vi "lijnvolgen.vi"() -> ()   [LabVIEW 2019]
uses:
  <vilib>/myRIO/Instrument Drivers/Onboard IO/AI/typedefs/AI Reference.ctl
  <vilib>/myRIO/Common/Instrument Driver Framework/Utilities/typedefs/myRIO Generic Hardware Reference.ctl
  <vilib>/myRIO/Common/Instrument Driver Framework/Utilities/typedefs/Hardware Version Enum.ctl
  <vilib>/myRIO/Common/Instrument Driver Framework/Utilities/typedefs/myRIO v1.0 Reference.ctl
  <vilib>/myRIO/Common/Instrument Driver Framework/Utilities/typedefs/Generic FPGA Reference.ctl
  <vilib>/myRIO/Common/Instrument Driver Framework/myRIO v1.0/AI/typedefs/AI Channels List.ctl
  <vilib>/myRIO/Common/Instrument Driver Framework/myRIO v1.0/AI/typedefs/AI Channels Enum.ctl
  <vilib>/myRIO/Common/Instrument Driver Framework/Utilities/typedefs/Analog Scaling Constants List.ctl
  <vilib>/myRIO/Common/Instrument Driver Framework/Utilities/typedefs/Analog Scaling Constants.ctl
  <vilib>/userDefined/High Color/nirio_resource_hc.ctl
  <vilib>/myRIO/Instrument Drivers/Onboard IO/AO/typedefs/AO Reference.ctl
  <vilib>/myRIO/Common/Instrument Driver Framework/myRIO v1.0/AO/typedefs/AO Channels List.ctl
  <vilib>/myRIO/Common/Instrument Driver Framework/myRIO v1.0/AO/typedefs/AO Channels Enum.ctl
  <vilib>/myRIO/Common/Instrument Driver Framework/Utilities/vis/Is FPGA Ref Available.vi
  <vilib>/myRIO/Common/Instrument Driver Framework/myRIO v1.0/AI/vis/myRIO v1.1 Open AI.vi
  <vilib>/myRIO/Instrument Drivers/Onboard IO/AI/vis/Read.vi
  <vilib>/myRIO/Common/Instrument Driver Framework/myRIO v1.0/AO/vis/myRIO v1.1 Open AO.vi
  <vilib>/myRIO/Instrument Drivers/Onboard IO/AO/vis/Write.vi
  <vilib>/myRIO/Common/Instrument Driver Framework/Utilities/vis/Validate Channels.vi
  <vilib>/myRIO/Common/Instrument Driver Framework/myRIO v1.0/AI/vis/myRIO v1.0 Reserve AI.vi
  <vilib>/myRIO/Common/Instrument Driver Framework/myRIO v1.0/AO/vis/myRIO v1.0 Reserve AO.vi
  <vilib>/myRIO/Common/Instrument Driver Framework/myRIO v1.0/AI/vis/myRIO v1.0 Build MUX Configuration AI.vi
  <vilib>/myRIO/Common/Instrument Driver Framework/myRIO v1.0/Resource Manager/vis/myRIO v1.0 Reserve Channel List.vi
  <vilib>/myRIO/Common/Instrument Driver Framework/myRIO v1.0/AO/vis/myRIO v1.0 Build MUX Configuration AO.vi
  <vilib>/myRIO/Common/Instrument Driver Framework/myRIO v1.0/Resource Manager/vis/myRIO v1.0 Reserve Channel.vi
  <vilib>/myRIO/Common/Instrument Driver Framework/myRIO v1.0/Resource Manager/vis/myRIO v1.0 Unreserve Channel.vi
  <vilib>/myRIO/Common/Instrument Driver Framework/myRIO v1.0/Resource Manager/vis/myRIO v1.0 Build Mutex Name.vi
  <vilib>/Utility/VariantDataType/GetNumericInfo.vi
  <vilib>/Utility/error.llb/Error Cluster From Error Code.vi
  <vilib>/myRIO/Common/Instrument Driver Framework/myRIO v1.0/myRIO v1.1 Open.vi
  <vilib>/myRIO/Common/Instrument Driver Framework/myRIO v1.0/AI/vis/myRIO v1.0 Get Scaling Constants AI.vi
  <vilib>/myRIO/Common/Instrument Driver Framework/Utilities/vis/IO Manager.vi
  <vilib>/myRIO/Common/Instrument Driver Framework/Utilities/vis/Configuration Manager.vi
  <vilib>/myRIO/Common/Instrument Driver Framework/myRIO v1.0/myRIO v1.0 Close.vi
  <vilib>/myRIO/Common/Instrument Driver Framework/myRIO v1.0/AI/vis/myRIO v1.0 Read AI.vi
  <vilib>/myRIO/Common/Instrument Driver Framework/myRIO v1.0/AO/vis/myRIO v1.0 Get Scaling Constants AO.vi
  <vilib>/myRIO/Common/Instrument Driver Framework/myRIO v1.0/AO/vis/myRIO v1.0 Write AO.vi
  <vilib>/myRIO/Express VI/Onboard IO/AI/AI Express VI.xnode
  <vilib>/myRIO/Instrument Drivers/Onboard IO/AI/vis/myRIO AI Open.xnode
  <vilib>/myRIO/Express VI/Onboard IO/AO/AO Express VI.xnode
  <vilib>/myRIO/Instrument Drivers/Onboard IO/AO/vis/myRIO AO Open.xnode
  <vilib>/myRIO/Instrument Drivers/Onboard IO/AO/AO.lvlib
  <vilib>/myRIO/Instrument Drivers/Onboard IO/AI/AI.lvlib
panel:
  in  "Boolean":bool
  out "Numeric 4":i32
  out "analoog":dbl[](array[numeric])
  out "Array 3":i32[](array[numeric])
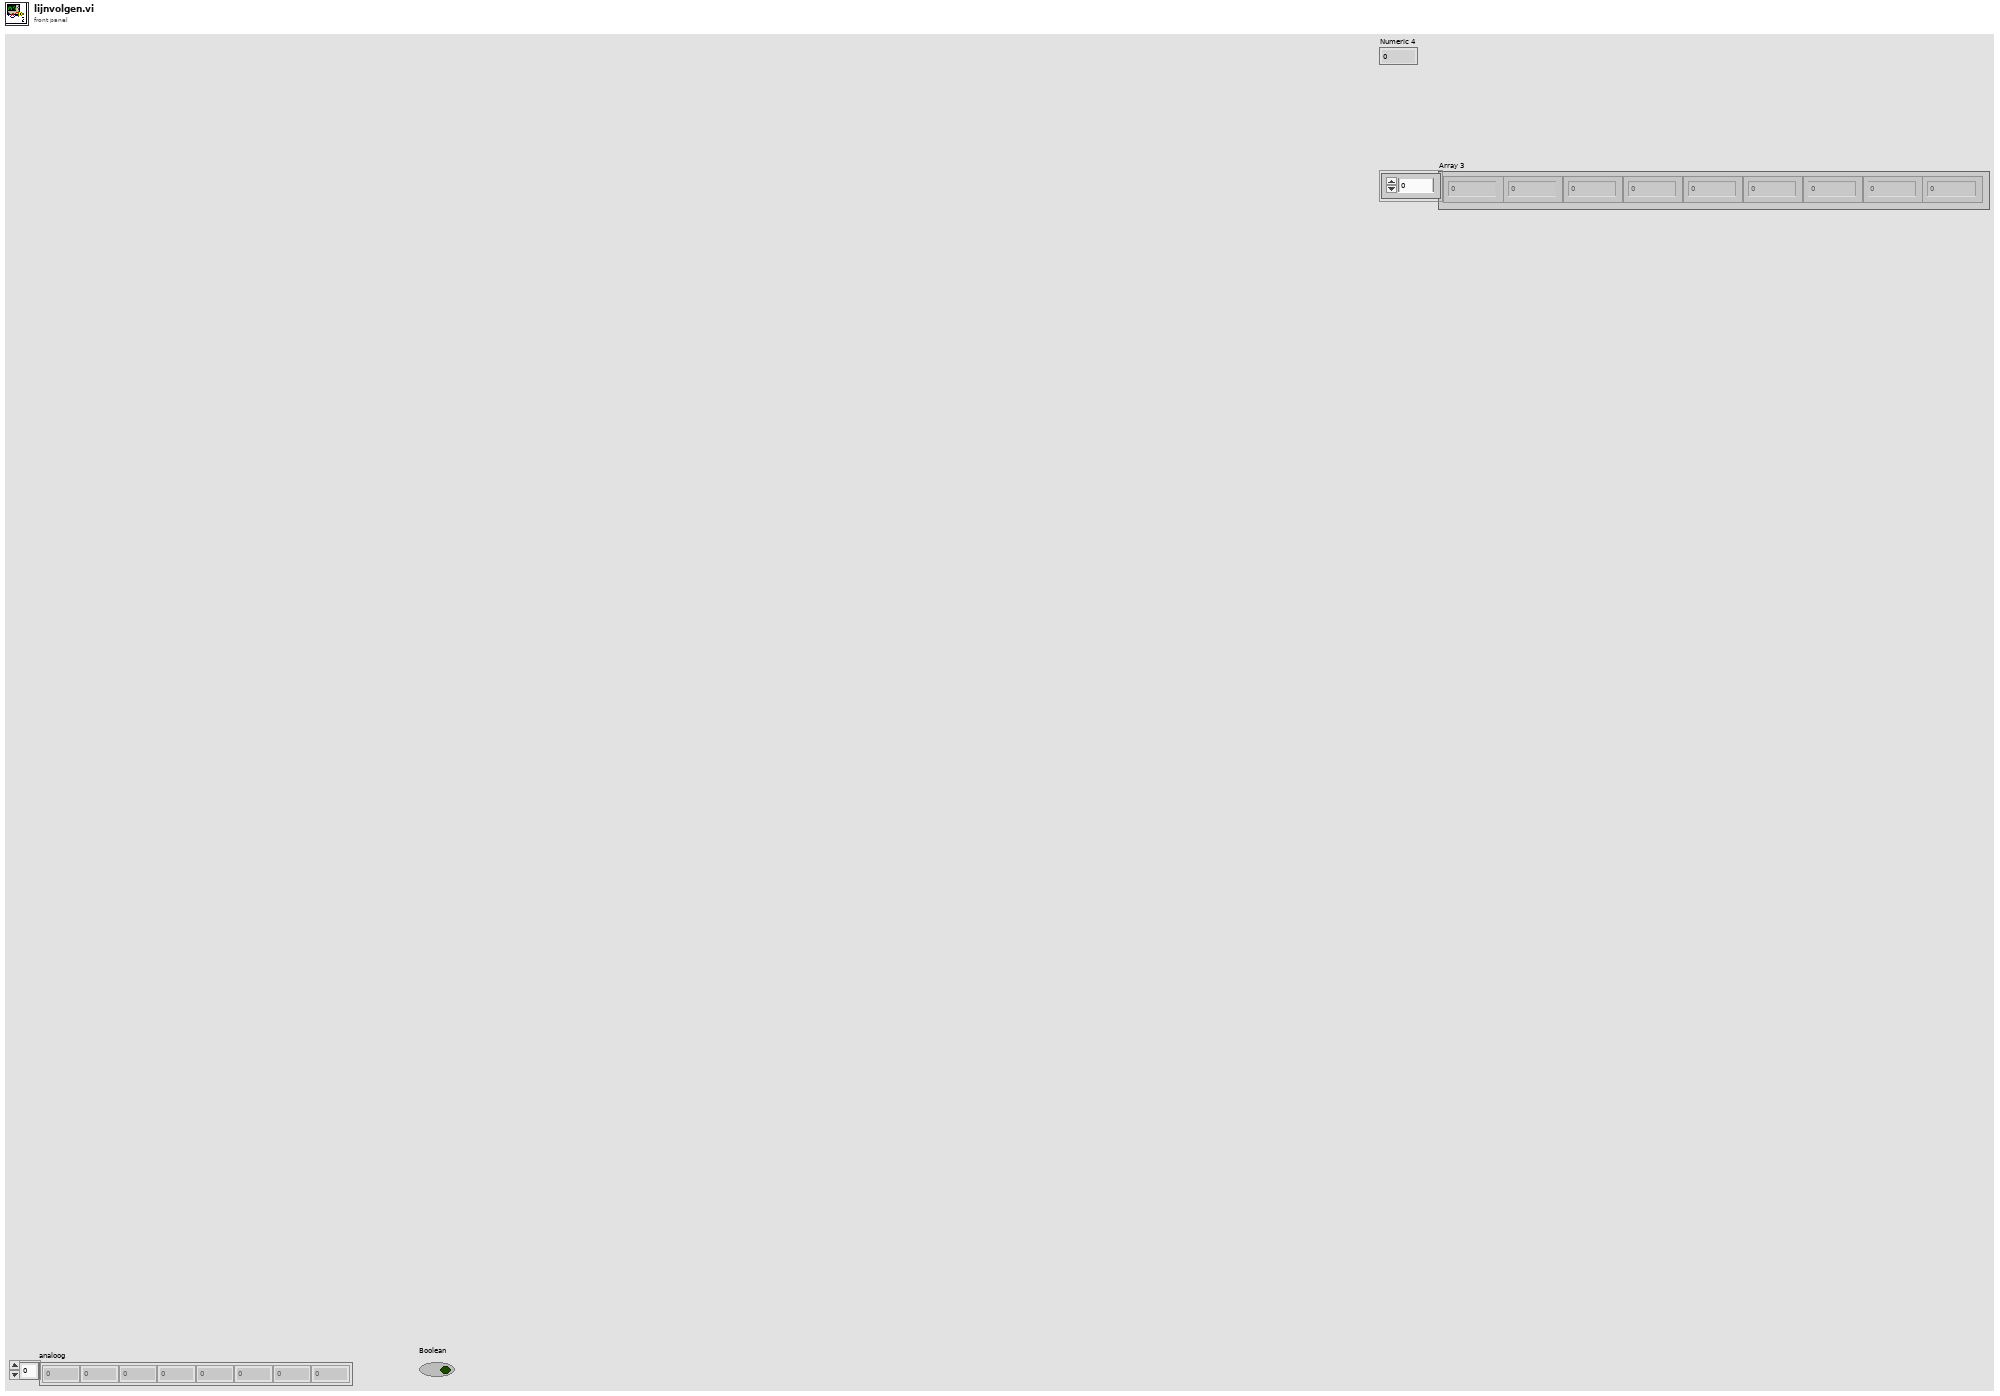
[diagram p1: front panel]
types:
  T1 = typedef "AO.lvlib/AO Reference.ctl" = cluster{"myRIO Reference":T2, "AO Channel List":T6, "AO Scaling Constant List":T8}
  T2 = typedef "myRIO Generic Hardware Reference.ctl" = cluster{"myRIO Model":T3, "myRIO Hardware Reference":T4}
  T3 = typedef "Hardware Version Enum.ctl" = enum16{"Unknown", "myRIO-1900", "myRIO-1950", "roboRIO", "NI ELVIS RIO CM", "ELVIS III"}
  T4 = typedef "myRIO v1.0 Reference.ctl" = cluster{"Generic FPGA Reference":T5, "Allow multiple opens":bool}
  T5 = typedef "Generic FPGA Reference.ctl" = refnum<k20>
  T6 = typedef "AO Channels List.ctl" = T7[]
  T7 = typedef "AO Channels Enum.ctl" = enum16{"Not Connected", "AudioOut/Left", "AudioOut/Right", "C/AO0", "C/AO1", "A/AO0", "A/AO1", "B/AO0", "B/AO1"}
  T8 = typedef "Analog Scaling Constants List.ctl" = T9[]
  T9 = typedef "Analog Scaling Constants.ctl" = cluster{"LSB Weight (Volts)":dbl, "Offset (Volts)":dbl, "Signed?":bool}
  T10 = typedef "nirio_resource_hc.ctl" = tag
  T11 = typedef "AI.lvlib/AI Reference.ctl" = cluster{"myRIO Reference":T2, "AI Channels List":T12, "AI Scaling Constants List":T8}
  T12 = typedef "AI Channels List.ctl" = T13[]
  T13 = typedef "AI Channels Enum.ctl" = enum16{"Not Connected", "AudioIn/Left", "AudioIn/Right", "C/AI0", "C/AI1", "A/AI0", "A/AI1", "A/AI2", "A/AI3", "A/AI4", "A/AI5", "A/AI6", "A/AI7", "B/AI0", "B/AI1", "B/AI2", "B/AI3", "B/AI4", "B/AI5", "B/AI6", "B/AI7", "AI/AI0", "AI/AI1", "AI/AI2", "AI/AI3", "A/AI0 (DIFF)", "A/AI1 (DIFF)", "A/AI2 (DIFF)", "A/AI3 (DIFF)", "B/AI0 (DIFF)", "B/AI1 (DIFF)", "B/AI2 (DIFF)", "B/AI3 (DIFF)"}
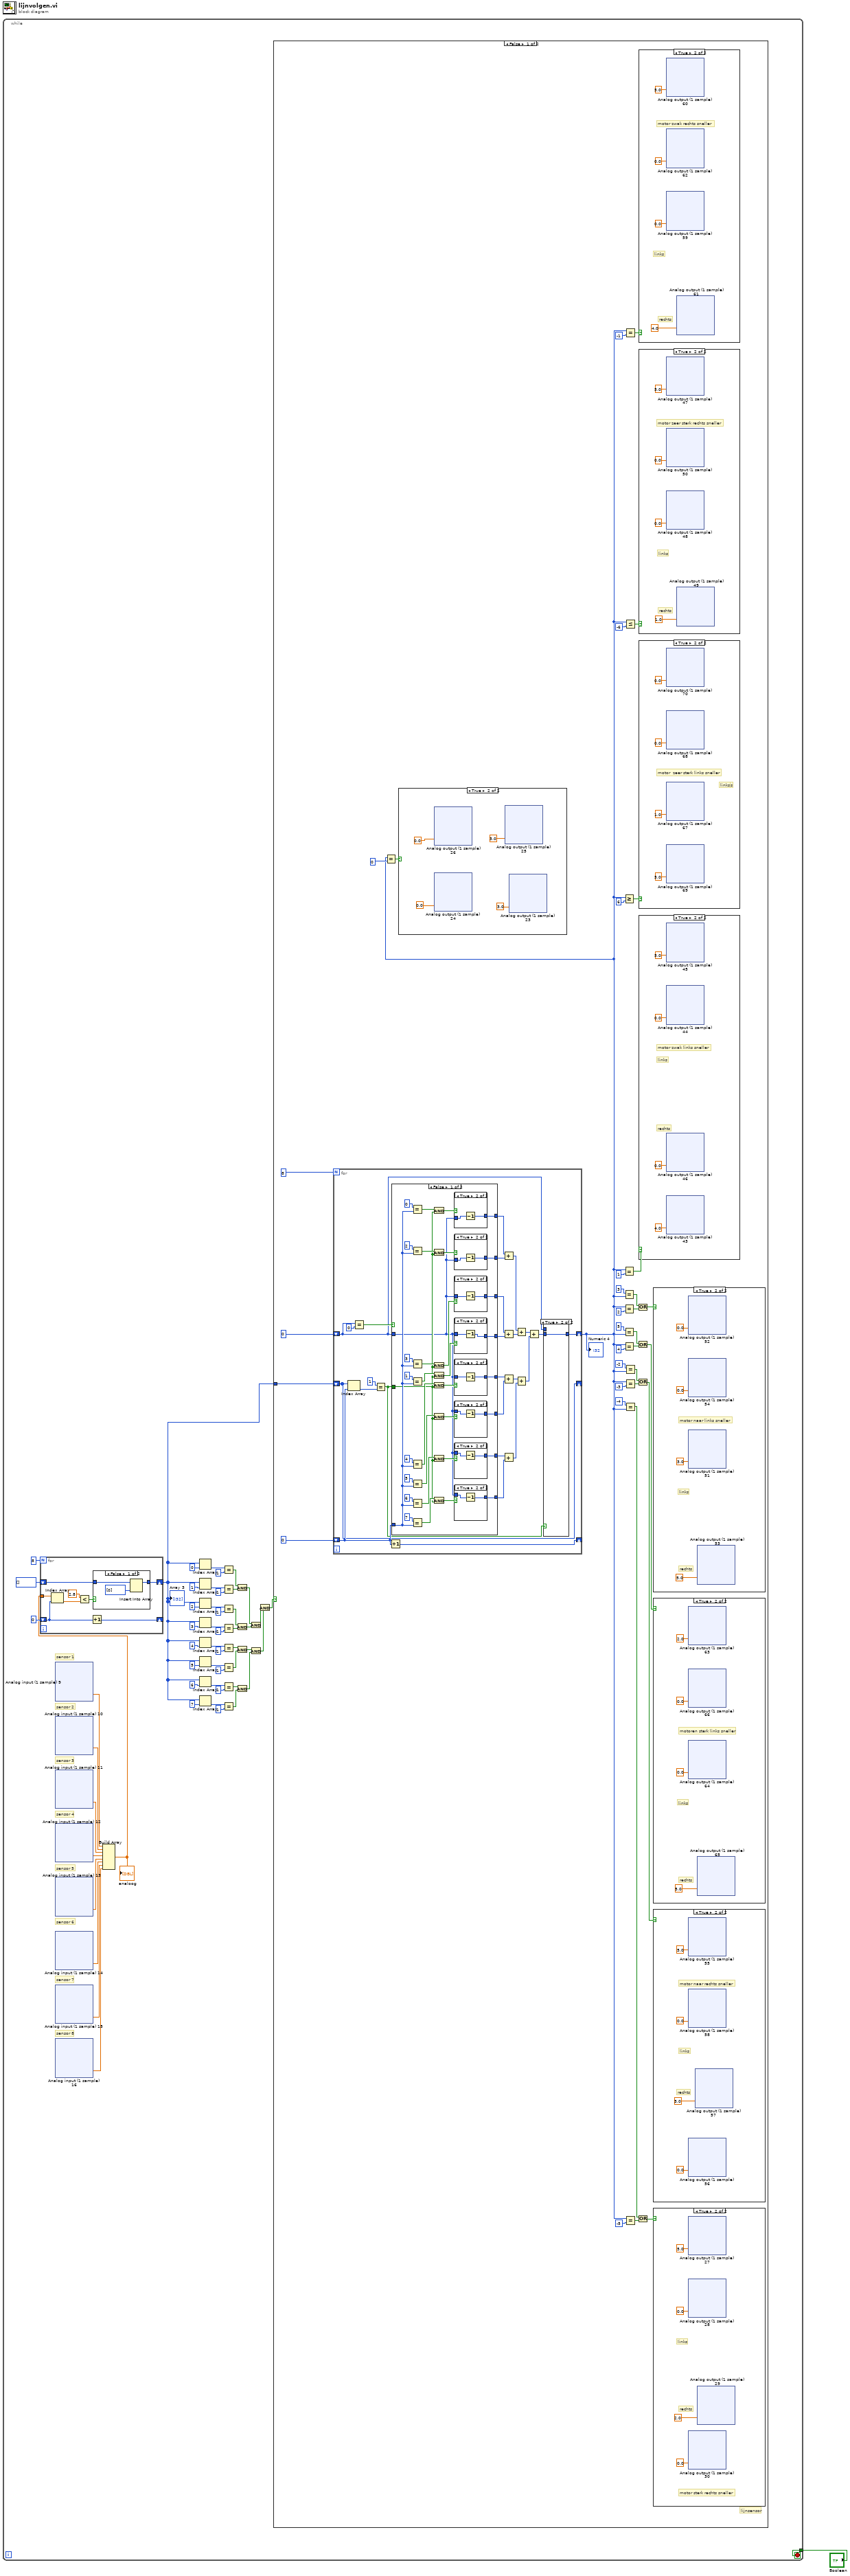
[diagram p0: block diagram]
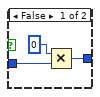
[diagram p12: hidden frame]
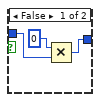
[diagram p13: hidden frame]
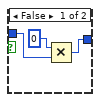
[diagram p14: hidden frame]
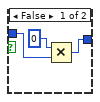
[diagram p15: hidden frame]
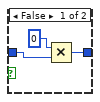
[diagram p16: hidden frame]
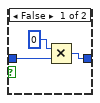
[diagram p17: hidden frame]
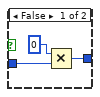
[diagram p18: hidden frame]
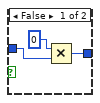
[diagram p19: hidden frame]
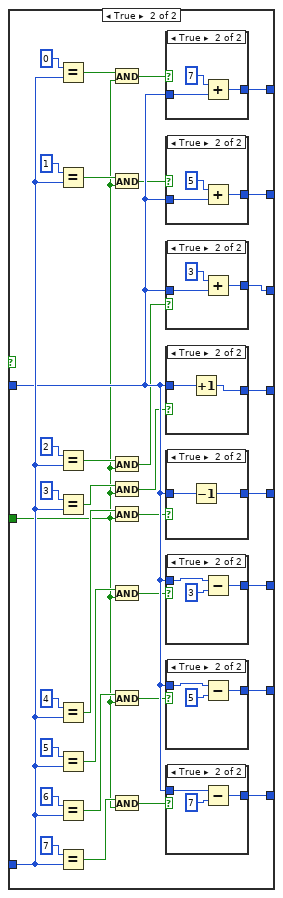
[diagram p20: hidden frame]
diagram:
  n1 = while {
    tunnel: "Boolean" -> [w2]
    stop <- w2 stop-if-true
    # "sensor 8"
    # "sensor 7"
    # "sensor 6"
    # "sensor 5"
    # "sensor 4"
    # "sensor 3"
    # "sensor 2"
    # "sensor 1"
    n2 = xnode "Analog input (1 sample) 9"() -> ("A/AI3 (Pin 9)"=w6:dbl)  [unwired: 1 in, 1 out]
    n3 = xnode "Analog input (1 sample) 10"() -> ("A/AI2 (Pin 7)"=w7:dbl)  [unwired: 1 in, 1 out]
    n4 = xnode "Analog input (1 sample) 11"() -> ("A/AI1 (Pin 5)"=w8:dbl)  [unwired: 1 in, 1 out]
    n5 = xnode "Analog input (1 sample) 12"() -> ("A/AI0 (Pin 3)"=w9:dbl)  [unwired: 1 in, 1 out]
    n6 = xnode "Analog input (1 sample) 13"() -> ("B/AI3 (Pin 9)"=w10:dbl)  [unwired: 1 in, 1 out]
    n7 = xnode "Analog input (1 sample) 14"() -> ("B/AI2 (Pin 7)"=w11:dbl)  [unwired: 1 in, 1 out]
    n8 = xnode "Analog input (1 sample) 15"() -> ("A/AI1 (Pin 5)"=w12:dbl)  [unwired: 1 in, 1 out]
    n9 = xnode "Analog input (1 sample) 16"() -> ("B/AI0 (Pin 3)"=w13:dbl)  [unwired: 1 in, 1 out]
    n10 = Build Array(w6, w7, w8, w9, w10, w11, w12, w13) -> (w5:dbl[])
    "analoog" <- w5
    n11 = for {
      N: 8 -> [_]
      shift-right: [w2095] -> w3
      shift-left: i32[] [] -> [w2096]
      shift-right: [w2092] -> _
      shift-left: 0 -> [w2091]
      tunnel: w5 -> [w2089]
      n12 = Index Array(array=w2089, index=w2091) -> (element=w2090:dbl)
      n13 = Less?(x=2.8, y=w2090) -> (x < y?=w2094:bool)
      n14 = Increment(x=w2091) -> (x+1=w2092:i32)
      n15 = case shown="False" w2094 {
        tunnel: w2096 -> [w2098 w2100]
        tunnel: [w2099 w2102] -> w2095
        frame False {
          n16 = Insert Into Array(array=w2098, new element=i32[] [0]) -> (w2099:i32[])  [unwired: 1 in]
        }
        frame True {
          n17 = Insert Into Array(array=w2100, new element=i32[] [1, 1]) -> (w2102:i32[])  [unwired: 1 in]
        }
      }
    }
    "Array 3" <- w3
    n18 = Index Array(array=w3, index=0) -> (element=w35:i32)
    n19 = Index Array(array=w3, index=1) -> (element=w14:i32)
    n20 = Index Array(array=w3, index=2) -> (element=w20:i32)
    n21 = Index Array(array=w3, index=3) -> (element=w17:i32)
    n22 = Index Array(array=w3, index=4) -> (element=w23:i32)
    n23 = Index Array(array=w3, index=5) -> (element=w26:i32)
    n24 = Index Array(array=w3, index=6) -> (element=w29:i32)
    n25 = Index Array(array=w3, index=7) -> (element=w32:i32)
    n26 = Equal?(x=w35, y=1) -> (x = y?=w38:bool)
    n27 = Equal?(x=w14, y=1) -> (x = y?=w39:bool)
    n28 = Equal?(x=w20, y=1) -> (x = y?=w40:bool)
    n29 = Equal?(x=w17, y=1) -> (x = y?=w41:bool)
    n30 = Equal?(x=w23, y=1) -> (x = y?=w42:bool)
    n31 = Equal?(x=w26, y=1) -> (x = y?=w43:bool)
    n32 = Equal?(x=w29, y=1) -> (x = y?=w44:bool)
    n33 = Equal?(x=w32, y=1) -> (x = y?=w45:bool)
    n34 = And(x=w38, y=w39) -> (x .and. y?=w46:bool)
    n35 = And(x=w40, y=w41) -> (x .and. y?=w47:bool)
    n36 = And(x=w42, y=w43) -> (x .and. y?=w48:bool)
    n37 = And(x=w44, y=w45) -> (x .and. y?=w49:bool)
    n38 = And(x=w46, y=w47) -> (x .and. y?=w50:bool)
    n39 = And(x=w48, y=w49) -> (x .and. y?=w51:bool)
    n40 = And(x=w50, y=w51) -> (x .and. y?=w4:bool)
    n41 = case shown="False" w4 {
      tunnel: w3 -> [w55 _]
      frame False {
        # "lijnsensor"
        n42 = for {
          N: 8 -> [_]
          shift-right: [w1468] -> _
          shift-left: 0 -> [w1482]
          shift-right: [w1460] -> w56
          shift-left: 0 -> [w1461]
          shift-right: [w1473] -> _
          shift-left: w55 -> [w1473]
          n43 = Index Array(array=w1473, index=w1482) -> (element=w1472:i32)
          n44 = Equal?(x=w1461, y=0) -> (x = y?=w1469:bool)
          n45 = Equal?(x=1, y=w1472) -> (x = y?=w1459:bool)
          n46 = Increment(x=w1482) -> (x+1=w1468:i32)
          n47 = case shown="False" w1469 {
            tunnel: w1482 -> [w1492 w1578]
            tunnel: [w1486 w1577] -> w1481
            tunnel: [w1493 w1576] -> w1480
            tunnel: [w1494 w1575] -> w1479
            tunnel: [w1495 w1574] -> w1478
            tunnel: w1461 -> [w1485 w1573]
            tunnel: w1459 -> [w1491 w1564]
            tunnel: [w1489 w1563] -> w1467
            tunnel: [w1490 w1562] -> w1466
            tunnel: [w1487 w1561] -> w1464
            tunnel: [w1488 w1560] -> w1463
            frame False {
              n48 = Equal?(x=0, y=w1492) -> (x = y?=w1512:bool)
              n49 = Equal?(x=2, y=w1492) -> (x = y?=w1518:bool)
              n50 = Equal?(x=3, y=w1492) -> (x = y?=w1519:bool)
              n51 = Equal?(x=1, y=w1492) -> (x = y?=w1504:bool)
              n52 = Equal?(x=4, y=w1492) -> (x = y?=w1516:bool)
              n53 = Equal?(x=5, y=w1492) -> (x = y?=w1517:bool)
              n54 = Equal?(x=6, y=w1492) -> (x = y?=w1515:bool)
              n55 = Equal?(x=7, y=w1492) -> (x = y?=w1514:bool)
              n56 = And(x=w1512, y=w1491) -> (x .and. y?=w1496:bool)
              n57 = And(x=w1518, y=w1491) -> (x .and. y?=w1498:bool)
              n58 = And(x=w1519, y=w1491) -> (x .and. y?=w1499:bool)
              n59 = And(x=w1504, y=w1491) -> (x .and. y?=w1497:bool)
              n60 = And(x=w1516, y=w1491) -> (x .and. y?=w1500:bool)
              n61 = And(x=w1517, y=w1491) -> (x .and. y?=w1501:bool)
              n62 = And(x=w1515, y=w1491) -> (x .and. y?=w1502:bool)
              n63 = And(x=w1514, y=w1491) -> (x .and. y?=w1503:bool)
              n64 = case shown="True" w1496 {
                tunnel: [w1521 w1524] -> w1490
                tunnel: w1485 -> [w1520 w1523]
                frame False {
                  n65 = Multiply(x=0, y=w1520) -> (x*y=w1521:i32)
                }
                frame True {
                  n66 = Decrement(x=w1523) -> (x-1=w1524:i32)
                }
              }
              n67 = case shown="True" w1498 {
                tunnel: [w1552 w1553] -> w1489
                tunnel: w1485 -> [w1551 w1554]
                frame False {
                  n68 = Multiply(x=0, y=w1551) -> (x*y=w1552:i32)
                }
                frame True {
                  n69 = Decrement(x=w1554) -> (x-1=w1553:i32)
                }
              }
              n70 = case shown="True" w1499 {
                tunnel: [w1546 w1549] -> w1488
                tunnel: w1485 -> [w1545 w1548]
                frame False {
                  n71 = Multiply(x=0, y=w1545) -> (x*y=w1546:i32)
                }
                frame True {
                  n72 = Decrement(x=w1548) -> (x-1=w1549:i32)
                }
              }
              n73 = case shown="True" w1497 {
                tunnel: [w1556 w1559] -> w1487
                tunnel: w1485 -> [w1555 w1558]
                frame False {
                  n74 = Multiply(x=0, y=w1555) -> (x*y=w1556:i32)
                }
                frame True {
                  n75 = Decrement(x=w1558) -> (x-1=w1559:i32)
                }
              }
              n76 = case shown="True" w1500 {
                tunnel: [w1541 w1544] -> w1486
                tunnel: w1485 -> [w1540 w1543]
                frame False {
                  n77 = Multiply(x=0, y=w1540) -> (x*y=w1541:i32)
                }
                frame True {
                  n78 = Decrement(x=w1543) -> (x-1=w1544:i32)
                }
              }
              n79 = case shown="True" w1501 {
                tunnel: [w1531 w1534] -> w1493
                tunnel: w1485 -> [w1530 w1533]
                frame False {
                  n80 = Multiply(x=0, y=w1530) -> (x*y=w1531:i32)
                }
                frame True {
                  n81 = Decrement(x=w1533) -> (x-1=w1534:i32)
                }
              }
              n82 = case shown="True" w1502 {
                tunnel: [w1536 w1539] -> w1494
                tunnel: w1485 -> [w1535 w1538]
                frame False {
                  n83 = Multiply(x=0, y=w1535) -> (x*y=w1536:i32)
                }
                frame True {
                  n84 = Decrement(x=w1538) -> (x-1=w1539:i32)
                }
              }
              n85 = case shown="True" w1503 {
                tunnel: [w1525 w1529] -> w1495
                tunnel: w1485 -> [w1526 w1528]
                frame False {
                  n86 = Multiply(x=0, y=w1526) -> (x*y=w1525:i32)
                }
                frame True {
                  n87 = Decrement(x=w1528) -> (x-1=w1529:i32)
                }
              }
            }
            frame True {
              n88 = Equal?(x=0, y=w1578) -> (x = y?=w1587:bool)
              n89 = Equal?(x=1, y=w1578) -> (x = y?=w1579:bool)
              n90 = Equal?(x=2, y=w1578) -> (x = y?=w1593:bool)
              n91 = Equal?(x=3, y=w1578) -> (x = y?=w1594:bool)
              n92 = Equal?(x=4, y=w1578) -> (x = y?=w1591:bool)
              n93 = Equal?(x=5, y=w1578) -> (x = y?=w1592:bool)
              n94 = Equal?(x=6, y=w1578) -> (x = y?=w1590:bool)
              n95 = Equal?(x=7, y=w1578) -> (x = y?=w1589:bool)
              n96 = And(x=w1587, y=w1564) -> (x .and. y?=w1565:bool)
              n97 = And(x=w1579, y=w1564) -> (x .and. y?=w1566:bool)
              n98 = And(x=w1593, y=w1564) -> (x .and. y?=w1567:bool)
              n99 = And(x=w1594, y=w1564) -> (x .and. y?=w1568:bool)
              n100 = And(x=w1591, y=w1564) -> (x .and. y?=w1569:bool)
              n101 = And(x=w1592, y=w1564) -> (x .and. y?=w1570:bool)
              n102 = And(x=w1590, y=w1564) -> (x .and. y?=w1571:bool)
              n103 = And(x=w1589, y=w1564) -> (x .and. y?=w1572:bool)
              n104 = case shown="True" w1565 {
                tunnel: w1573 -> [w1595 w1599]
                tunnel: [w1596 w1598] -> w1562
                frame False {
                  n105 = Multiply(x=0, y=w1595) -> (x*y=w1596:i32)
                }
                frame True {
                  n106 = Add(x=7, y=w1599) -> (x+y=w1598:i32)
                }
              }
              n107 = case shown="True" w1566 {
                tunnel: w1573 -> [w1635 w1638]
                tunnel: [w1636 w1639] -> w1563
                frame False {
                  n108 = Multiply(x=0, y=w1635) -> (x*y=w1636:i32)
                }
                frame True {
                  n109 = Add(x=5, y=w1638) -> (x+y=w1639:i32)
                }
              }
              n110 = case shown="True" w1567 {
                tunnel: w1573 -> [w1629 w1633]
                tunnel: [w1630 w1632] -> w1560
                frame False {
                  n111 = Multiply(x=0, y=w1629) -> (x*y=w1630:i32)
                }
                frame True {
                  n112 = Add(x=3, y=w1633) -> (x+y=w1632:i32)
                }
              }
              n113 = case shown="True" w1568 {
                tunnel: w1573 -> [w1625 w1628]
                tunnel: [w1624 w1627] -> w1561
                frame False {
                  n114 = Multiply(x=0, y=w1625) -> (x*y=w1624:i32)
                }
                frame True {
                  n115 = Increment(x=w1628) -> (x+1=w1627:i32)
                }
              }
              n116 = case shown="True" w1569 {
                tunnel: w1573 -> [w1619 w1623]
                tunnel: [w1620 w1622] -> w1577
                frame False {
                  n117 = Multiply(x=0, y=w1619) -> (x*y=w1620:i32)
                }
                frame True {
                  n118 = Decrement(x=w1623) -> (x-1=w1622:i32)
                }
              }
              n119 = case shown="True" w1570 {
                tunnel: w1573 -> [w1608 w1610]
                tunnel: [w1607 w1612] -> w1576
                frame False {
                  n120 = Multiply(x=0, y=w1608) -> (x*y=w1607:i32)
                }
                frame True {
                  n121 = Subtract(x=w1610, y=3) -> (x-y=w1612:i32)
                }
              }
              n122 = case shown="True" w1571 {
                tunnel: w1573 -> [w1614 w1616]
                tunnel: [w1613 w1617] -> w1575
                frame False {
                  n123 = Multiply(x=0, y=w1614) -> (x*y=w1613:i32)
                }
                frame True {
                  n124 = Subtract(x=w1616, y=5) -> (x-y=w1617:i32)
                }
              }
              n125 = case shown="True" w1572 {
                tunnel: w1573 -> [w1601 w1604]
                tunnel: [w1602 w1605] -> w1574
                frame False {
                  n126 = Multiply(x=0, y=w1601) -> (x*y=w1602:i32)
                }
                frame True {
                  n127 = Subtract(x=w1604, y=7) -> (x-y=w1605:i32)
                }
              }
            }
          }
          n128 = Add(x=w1466, y=w1467) -> (x+y=w1465:i32)
          n129 = Add(x=w1463, y=w1464) -> (x+y=w1462:i32)
          n130 = Add(x=w1481, y=w1480) -> (x+y=w1476:i32)
          n131 = Add(x=w1479, y=w1478) -> (x+y=w1477:i32)
          n132 = Add(x=w1465, y=w1462) -> (x+y=w1475:i32)
          n133 = Add(x=w1476, y=w1477) -> (x+y=w1474:i32)
          n134 = Add(x=w1475, y=w1474) -> (x+y=w1458:i32)
          n135 = case shown="True" w1459 {
            tunnel: w1461 -> [w1483 _]
            tunnel: [w1483 w1484] -> w1460
            tunnel: w1458 -> [_ w1484]
            frame False {
            }
            frame True {
            }
          }
        }
        "Numeric 4" <- w56
        n136 = Equal?(x=w56, y=0) -> (x = y?=w58:bool)
        n137 = case shown="True" w58 {
          frame False {
          }
          frame True {
            n138 = xnode "Analog output (1 sample) 24"("B/AO0 (Pin 2)"=0.0) -> ()  [unwired: 1 in, 1 out]
            n139 = xnode "Analog output (1 sample) 26"("A/AO0 (Pin 2)"=0.0) -> ()  [unwired: 1 in, 1 out]
            n140 = xnode "Analog output (1 sample) 25"("A/AO1 (Pin 4)"=3.0) -> ()  [unwired: 1 in, 1 out]
            n141 = xnode "Analog output (1 sample) 23"("B/AO1 (Pin 4)"=3.0) -> ()  [unwired: 1 in, 1 out]
          }
        }
        n142 = Greater Or Equal?(x=w56, y=6) -> (x >= y?=w84:bool)
        n143 = Equal?(x=w56, y=1) -> (x = y?=w85:bool)
        n144 = Equal?(x=3, y=w56) -> (x = y?=w75:bool)
        n145 = Equal?(x=w56, y=2) -> (x = y?=w76:bool)
        n146 = Equal?(x=5, y=w56) -> (x = y?=w79:bool)
        n147 = Equal?(x=w56, y=4) -> (x = y?=w80:bool)
        n148 = Equal?(x=w56, y=-1) -> (x = y?=w63:bool)
        n149 = Less Or Equal?(x=w56, y=-6) -> (x <= y?=w61:bool)
        n150 = Equal?(x=-2, y=w56) -> (x = y?=w69:bool)
        n151 = Equal?(x=w56, y=-3) -> (x = y?=w70:bool)
        n152 = Equal?(x=-4, y=w56) -> (x = y?=w65:bool)
        n153 = Equal?(x=w56, y=-5) -> (x = y?=w66:bool)
        n154 = Or(x=w75, y=w76) -> (x .or. y?=w73:bool)
        n155 = Or(x=w79, y=w80) -> (x .or. y?=w81:bool)
        n156 = Or(x=w69, y=w70) -> (x .or. y?=w62:bool)
        n157 = Or(x=w65, y=w66) -> (x .or. y?=w59:bool)
        n158 = case shown="True" w63 {
          frame False {
          }
          frame True {
            # "rechts"
            # "links"
            # "motor zwak rechts sneller"
            n159 = xnode "Analog output (1 sample) 60"("B/AO1 (Pin 4)"=5.0) -> ()  [unwired: 1 in, 1 out]
            n160 = xnode "Analog output (1 sample) 62"("A/AO0 (Pin 2)"=0.0) -> ()  [unwired: 1 in, 1 out]
            n161 = xnode "Analog output (1 sample) 59"("B/AO0 (Pin 2)"=0.0) -> ()  [unwired: 1 in, 1 out]
            n162 = xnode "Analog output (1 sample) 61"("A/AO1 (Pin 4)"=4.0) -> ()  [unwired: 1 in, 1 out]
          }
        }
        n163 = case shown="True" w61 {
          frame False {
          }
          frame True {
            # "rechts"
            # "links"
            # "motor zeer sterk rechts sneller"
            n164 = xnode "Analog output (1 sample) 47"("B/AO1 (Pin 4)"=5.0) -> ()  [unwired: 1 in, 1 out]
            n165 = xnode "Analog output (1 sample) 50"("A/AO0 (Pin 2)"=0.0) -> ()  [unwired: 1 in, 1 out]
            n166 = xnode "Analog output (1 sample) 48"("B/AO0 (Pin 2)"=0.0) -> ()  [unwired: 1 in, 1 out]
            n167 = xnode "Analog output (1 sample) 49"("A/AO1 (Pin 4)"=1.0) -> ()  [unwired: 1 in, 1 out]
          }
        }
        n168 = case shown="True" w84 {
          frame False {
          }
          frame True {
            # "rechts"
            # "links"
            # "motor  zeer sterk links sneller"
            n169 = xnode "Analog output (1 sample) 70"("A/AO0 (Pin 2)"=0.0) -> ()  [unwired: 1 in, 1 out]
            n170 = xnode "Analog output (1 sample) 68"("B/AO0 (Pin 2)"=0.0) -> ()  [unwired: 1 in, 1 out]
            n171 = xnode "Analog output (1 sample) 67"("B/AO1 (Pin 4)"=1.0) -> ()  [unwired: 1 in, 1 out]
            n172 = xnode "Analog output (1 sample) 69"("A/AO1 (Pin 4)"=5.0) -> ()  [unwired: 1 in, 1 out]
          }
        }
        n173 = case shown="True" w85 {
          frame False {
          }
          frame True {
            # "rechts"
            # "links"
            # "motor zwak links sneller"
            n174 = xnode "Analog output (1 sample) 45"("A/AO1 (Pin 4)"=5.0) -> ()  [unwired: 1 in, 1 out]
            n175 = xnode "Analog output (1 sample) 44"("B/AO0 (Pin 2)"=0.0) -> ()  [unwired: 1 in, 1 out]
            n176 = xnode "Analog output (1 sample) 46"("A/AO0 (Pin 2)"=0.0) -> ()  [unwired: 1 in, 1 out]
            n177 = xnode "Analog output (1 sample) 43"("B/AO1 (Pin 4)"=4.0) -> ()  [unwired: 1 in, 1 out]
          }
        }
        n178 = case shown="True" w73 {
          frame False {
          }
          frame True {
            # "rechts"
            # "links"
            # "motor naar links sneller"
            n179 = xnode "Analog output (1 sample) 52"("B/AO0 (Pin 2)"=0.0) -> ()  [unwired: 1 in, 1 out]
            n180 = xnode "Analog output (1 sample) 54"("A/AO0 (Pin 2)"=0.0) -> ()  [unwired: 1 in, 1 out]
            n181 = xnode "Analog output (1 sample) 51"("B/AO1 (Pin 4)"=3.0) -> ()  [unwired: 1 in, 1 out]
            n182 = xnode "Analog output (1 sample) 53"("A/AO1 (Pin 4)"=5.0) -> ()  [unwired: 1 in, 1 out]
          }
        }
        n183 = case shown="True" w81 {
          frame False {
          }
          frame True {
            # "rechts"
            # "links"
            # "motoren sterk links sneller"
            n184 = xnode "Analog output (1 sample) 63"("B/AO1 (Pin 4)"=2.0) -> ()  [unwired: 1 in, 1 out]
            n185 = xnode "Analog output (1 sample) 66"("A/AO0 (Pin 2)"=0.0) -> ()  [unwired: 1 in, 1 out]
            n186 = xnode "Analog output (1 sample) 64"("B/AO0 (Pin 2)"=0.0) -> ()  [unwired: 1 in, 1 out]
            n187 = xnode "Analog output (1 sample) 65"("A/AO1 (Pin 4)"=5.0) -> ()  [unwired: 1 in, 1 out]
          }
        }
        n188 = case shown="True" w62 {
          frame False {
          }
          frame True {
            # "rechts"
            # "links"
            # "motor naar rechts sneller"
            n189 = xnode "Analog output (1 sample) 55"("B/AO1 (Pin 4)"=5.0) -> ()  [unwired: 1 in, 1 out]
            n190 = xnode "Analog output (1 sample) 58"("A/AO0 (Pin 2)"=0.0) -> ()  [unwired: 1 in, 1 out]
            n191 = xnode "Analog output (1 sample) 56"("B/AO0 (Pin 2)"=0.0) -> ()  [unwired: 1 in, 1 out]
            n192 = xnode "Analog output (1 sample) 57"("A/AO1 (Pin 4)"=3.0) -> ()  [unwired: 1 in, 1 out]
          }
        }
        n193 = case shown="True" w59 {
          frame False {
          }
          frame True {
            # "rechts"
            # "links"
            # "motor sterk rechts sneller"
            n194 = xnode "Analog output (1 sample) 27"("B/AO1 (Pin 4)"=5.0) -> ()  [unwired: 1 in, 1 out]
            n195 = xnode "Analog output (1 sample) 28"("B/AO0 (Pin 2)"=0.0) -> ()  [unwired: 1 in, 1 out]
            n196 = xnode "Analog output (1 sample) 30"("A/AO0 (Pin 2)"=0.0) -> ()  [unwired: 1 in, 1 out]
            n197 = xnode "Analog output (1 sample) 29"("A/AO1 (Pin 4)"=2.0) -> ()  [unwired: 1 in, 1 out]
          }
        }
      }
      frame True {
        n198 = xnode "Analog output (1 sample)"("A/AO0 (Pin 2)"=0) -> ()  [unwired: 1 in, 1 out]
        n199 = xnode "Analog output (1 sample) 3"("B/AO0 (Pin 2)"=0) -> ()  [unwired: 1 in, 1 out]
        n200 = xnode "Analog output (1 sample) 2"("A/AO1 (Pin 4)"=0) -> ()  [unwired: 1 in, 1 out]
        n201 = xnode "Analog output (1 sample) 4"("B/AO1 (Pin 4)"=0) -> ()  [unwired: 1 in, 1 out]
      }
    }
  }
